vi "x4_.vi"() -> ()   [LabVIEW 2014]
panel:
  in  "x4_":dbl
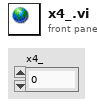
[diagram p1: front panel]
diagram:
